vi "Set Class Data.vi"(4 "Class name":string, 6 "Class versions":T1(array[cluster]), 7 "Object":refnum<class>, 8 "error in (no error)":errorcluster, 10 "Class default data":variant[](array[variant]), 11 "CConfig Variant Accessor in":refnum<class "CConfig Variant Accessor.lvclass">) -> (0 "error out":errorcluster, 3 "CConfig Variant Accessor out":refnum<class "CConfig Variant Accessor.lvclass">, 5 "Object (dup)":refnum<class>)   [LabVIEW 2013, in "CConfig Variant Accessor.lvclass"]
doc: "Copyright 2018, Carya Automatisering, Wiebe Walstra."
uses:
  CConfig Variant Accessor.lvclass
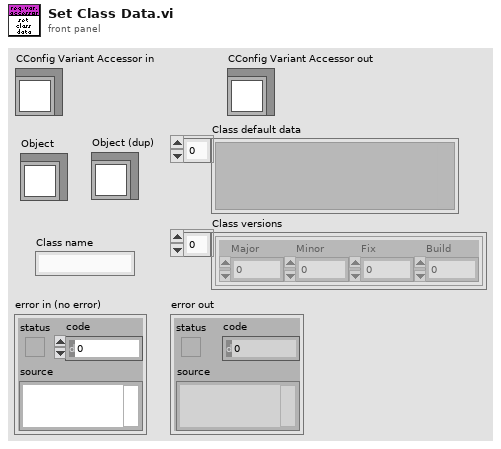
[diagram p1: front panel]
types:
  T1 = cluster{"Major":u16, "Minor":u16, "Fix":u16, "Build":u16}[]
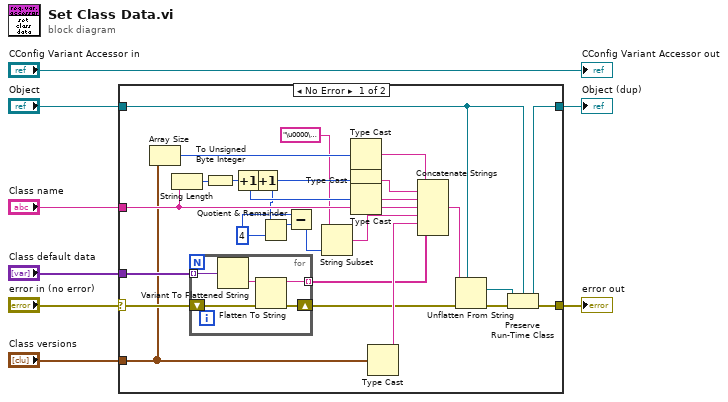
[diagram p0: block diagram]
diagram:
  n1 = case shown="No Error" "error in (no error)" {
    selector: "error in (no error)" -> [w21 w41]
    tunnel: [w16 w41] -> w7
    tunnel: "Object" -> [w19 w40]
    tunnel: [w18 w40] -> w4
    tunnel: "Class name" -> [w23 _]
    tunnel: "Class default data" -> [w22 _]
    tunnel: "Class versions" -> [w15 _]
    frame No Error {
      w12 = u8 4 ("y")
      n2 = Array Size(array=w15) -> (size(s)=w25:i32)
      n3 = String Length(string=w23) -> (length=w34:i32)
      n4 = for {
        tunnel: [w38] -> w27 mode=indexing
        tunnel: w22 -> [w37] mode=indexing
        shift-right: [w35] -> w24
        shift-left: w21 -> [w36]
        n5 = Variant To Flattened String(Variant=w37) -> (data string=w39:string)  [unwired: 1 out]
        n6 = Flatten To String(anything=w39, error in (no error)=w36) -> (data string=w38:string, error out=w35:errorcluster)  [unwired: 2 in, 1 out]
      }
      n7 = To Unsigned Byte Integer(number=w34) -> (unsigned 8bit integer=w30:u8)
      n8 = Increment(x=w30) -> (x+1=w33:u8)
      n9 = Increment(x=w33) -> (x+1=w14:u8)
      n10 = Quotient & Remainder(x=w14, y=w12) -> (x-y*floor(x/y)=w13:u8)  [unwired: 1 out]
      n11 = Subtract(x=w12, y=w13) -> (x-y=w11:u8)
      n12 = String Subset(string="\u0000\u0000\u0000", length (rest)=w11) -> (substring=w9:string)  [unwired: 1 in]
      n13 = Type Cast(x=w25) -> (*(type *) &x=w32:string)  [unwired: 1 in]
      n14 = Type Cast(x=w14) -> (*(type *) &x=w31:string)  [unwired: 1 in]
      n15 = Type Cast(x=w30) -> (*(type *) &x=w29:string)  [unwired: 1 in]
      n16 = Type Cast(x=w15) -> (*(type *) &x=w28:string)  [unwired: 1 in]
      n17 = Concatenate Strings(w32, w31, w29, w23, w9, w28, w27) -> (w26:string)
      n18 = Unflatten From String(type=w19, binary string=w26, error in (no error)=w24) -> (value=w20:refnum<class>, error out=w17:errorcluster)  [unwired: 2 in, 1 out]
      n19 = Preserve Run-Time Class(object in=w20, error in=w17, 2:w19) -> (object out=w18:refnum<class>, error out=w16:errorcluster)
    }
    frame Error {
    }
  }
  "error out" <- w7
  "Object (dup)" <- w4
  "CConfig Variant Accessor out" <- "CConfig Variant Accessor in"
